vi "Generator Test Bench.vi"() -> ()   [LabVIEW 2014]
uses:
  Controls/Gen Data.ctl
  Controls/NamedError.ctl
panel:
  out "String":string
  in  "Generator ON West":bool=TRUE
  out "Gen West":T1
  out "Gen Data West":T2 {"Alarms" format="%04x"}
  in  "Clear Error":bool
  in  "stop":bool
  # "0  Init          \n    1  Ready         \n    2  NotReady      \n    3  Prestart      \n    4  Cranking      \n    5  Pause         \n    6  Starting      \n    7  Running       \n    8  Loaded        \n    9  Soft unld     \n   10  Cooling       \n   11  Stop          \n   12  Shutdown      \n   13  Ventil        \n   14  EmergMan      \n   15  Cooldown      \n   16  Offload       \n   17  Soft load     \n   18  WaitStop      \n   19  Warming       \n   20  SDVentil"
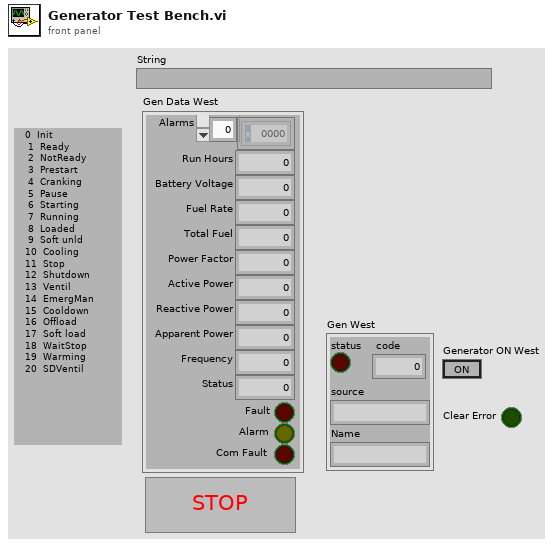
[diagram p1: front panel]
types:
  T1 = typedef "NamedError.ctl" = cluster{"status":bool, "code":i32, "source":string, "Name":string}
  T2 = typedef "Gen Data.ctl" = cluster{"Alarms":i16[], "Run Hours":dbl, "Battery Voltage":dbl, "Fuel Rate":dbl, "Total Fuel":dbl, "Power Factor":dbl, "Active Power":dbl, "Reactive Power":dbl, "Apparent Power":dbl, "Frequency":dbl, "Status":u16, "Fault":bool, "Alarm":bool, "Com Fault":bool}
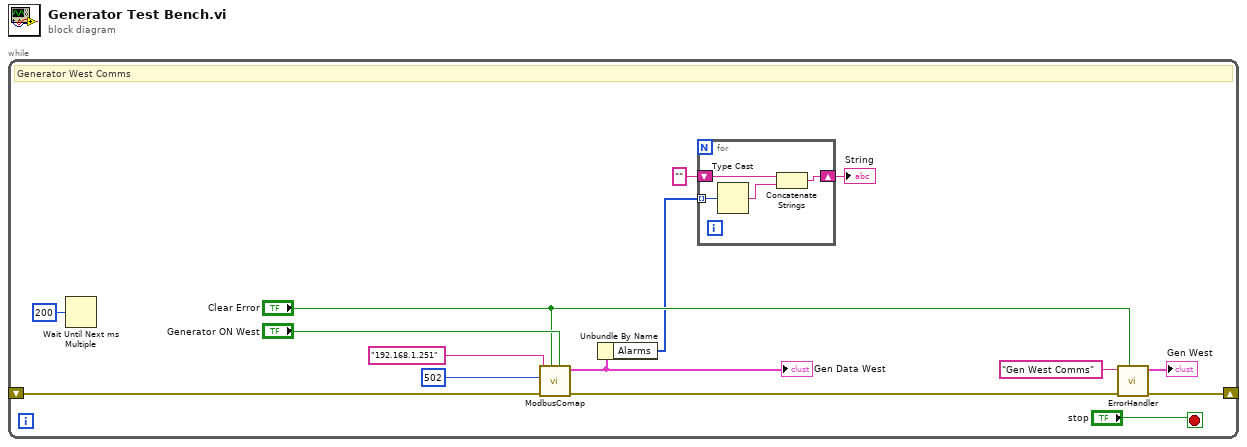
[diagram p0: block diagram]
diagram:
  n1 = while "Generator Comms" {
    shift-right: [w12] -> _
    shift-left: _ -> [w8]
    stop <- "stop" stop-if-true
    # "Generator West Comms"
    n2 = Wait Until Next ms Multiple(millisecond multiple=u32 200 ("milliseconds to wait")) -> ()  [unwired: 1 out]
    n3 = call "ModbusComap.vi"("Generator On"="Generator ON West", "Clear Alarms"="Clear Error", "Error In"=w8, "port (502)"=u16 502, "address"="192.168.1.251") -> ("Error Out"=w11:errorcluster, "Gen Data"=w3:T2)  [unwired: 3 in]
    "Gen Data West" <- w3
    n4 = Unbundle By Name(w3) -> ("Alarms"=w2:i16[])
    n5 = for {
      tunnel: w2 -> [w19] mode=indexing
      shift-right: [w18] -> w1
      shift-left: "" -> [w16]
      n6 = Type Cast(x=w19) -> (*(type *) &x=w17:string)  [unwired: 1 in]
      n7 = Concatenate Strings(w16, w17) -> (w18:string)
    }
    "String" <- w1
    n8 = call "ErrorHandler.vi"("Clear Error"="Clear Error", "Error In"=w11, "Name"="Gen West Comms") -> ("Error Out"=w12:errorcluster, "Named Error Out"=→"Gen West":T1)  [unwired: 5 in]
  }
